vi "InizializzaFile_funzioni_correttrici.vi"(10 "banco":i32=1) -> ()   [LabVIEW 2019]
uses:
  <vilib>/Utility/file.llb/Read Delimited Spreadsheet (string).vi
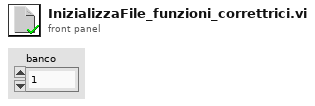
[diagram p1: front panel]
types:
  T1 = enum16{"open", "replace", "create", "open or create", "replace or create", "replace or create with confirmation"}
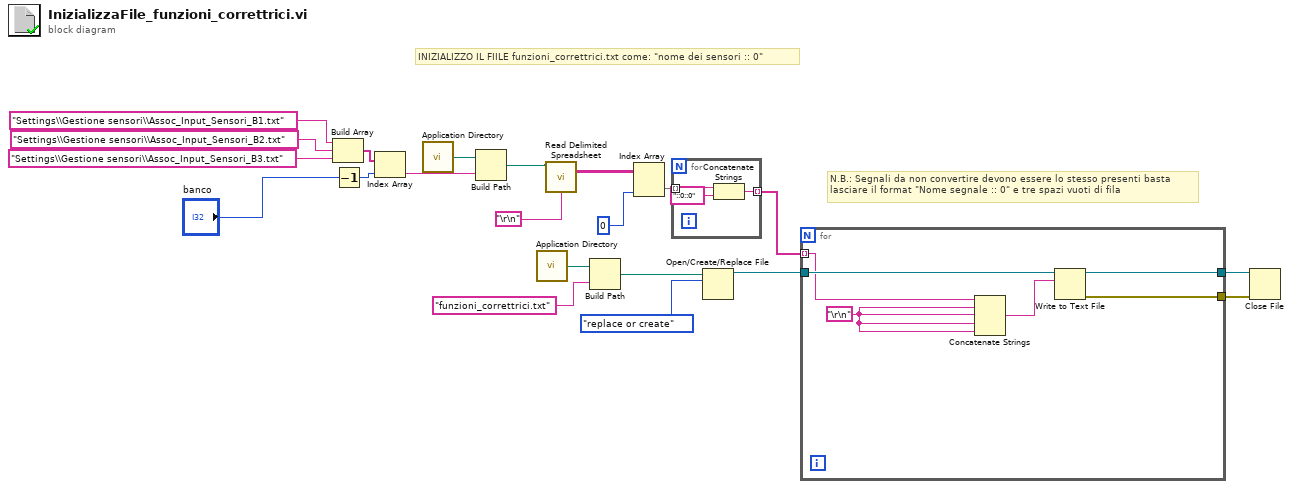
[diagram p0: block diagram]
diagram:
  # "INIZIALIZZO IL FIILE funzioni_correttrici.txt come: \"nome dei sensori :: 0\""
  # "N.B.: Segnali da non convertire devono essere lo stesso presenti basta \nlasciare il format \"Nome segnale :: 0\" e tre spazi vuoti di fila"
  n1 = Build Array("Settings\\Gestione sensori\\Assoc_Input_Sensori_B1.txt" ("name or relative path"), "Settings\\Gestione sensori\\Assoc_Input_Sensori_B2.txt" ("name or relative path"), "Settings\\Gestione sensori\\Assoc_Input_Sensori_B3.txt" ("name or relative path")) -> (w11:string[])
  n2 = Decrement(x="banco") -> (x-1=w10:i32)
  n3 = Index Array(array=w11, index=w10) -> (element=w8:string)
  n4 = call <vilib>:"Application Directory.vi"() -> ("Application Directory"=w9:path)
  n5 = Build Path(base path=w9, name or relative path=w8) -> (appended path=w6:path)
  n6 = call <vilib>:"Application Directory.vi"() -> ("Application Directory"=w20:path)
  n7 = call-poly <vilib>:"Read Delimited Spreadsheet.vi"("file path (dialog if empty)"=w6, "delimiter (\\t)"="\r\n" ("delimiter (\\t)")) -> ("all rows"=w4:string[][])  [unwired: 8 in, 5 out]
  n8 = Build Path(base path=w20, name or relative path="funzioni_correttrici.txt") -> (appended path=w19:path)
  n9 = Index Array(array=w4, index (col)=0 ("disabled index (col)")) -> (element=w2:string[])  [unwired: 1 in]
  n10 = for {
    tunnel: w2 -> [w24] mode=indexing
    tunnel: [w22] -> w1 mode=indexing
    n11 = Concatenate Strings(w24, "::0::0" ("string")) -> (w22:string)
  }
  n12 = Open/Create/Replace File(file path (use dialog)=w19, operation (0:open)=T1."replace or create") -> (refnum out=w17:refnum<file>)  [unwired: 4 in, 2 out]
  n13 = for {
    tunnel: w1 -> [w29] mode=indexing
    tunnel: w17 -> [w30]
    tunnel: [w26] -> w16
    tunnel: [w25] -> w15
    w28 = "\r\n"
    n14 = Concatenate Strings(w29, w28, w28, w28, w28) -> (w27:string)
    n15 = Write to Text File(file (use dialog)=w30, text=w27) -> (refnum out=w26:refnum<file>, error out=w25:errorcluster)  [unwired: 2 in, 1 out]
  }
  n16 = Close File(refnum=w16, error in=w15) -> ()  [unwired: 2 out]
